vi "Get Element.vi"(8 "error in":errorcluster, 10 "element name":string, 11 "cluster in":variant) -> (0 "error out":errorcluster, 2 "element":variant, 3 "cluster out":variant)   [LabVIEW 2020, in "PV Access.lvlib" / "PV Data.lvlib"]
uses:
  PV Data.lvlib
  <userlib>/_OpenG.lib/lvdata/lvdata.llb/openg_variant.lvlib
  <userlib>/_OpenG.lib/error/error.llb/openg_error.lvlib
  Error Codes.ctl
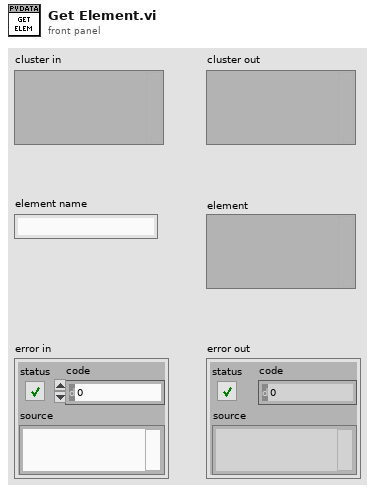
[diagram p1: front panel]
types:
  T1 = typedef "PV Access.lvlib/PV Data.lvlib/Error Codes.ctl" = i32
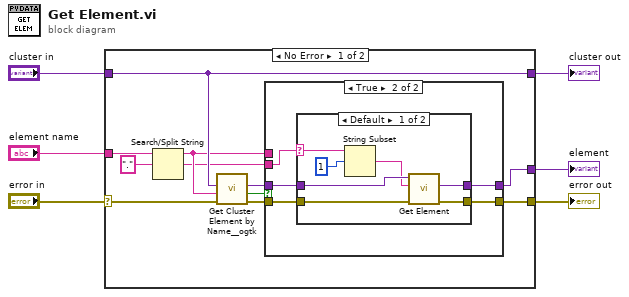
[diagram p0: block diagram]
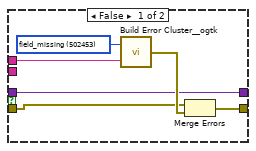
[diagram p2: hidden frame]
diagram:
  n1 = case shown="No Error" "error in" {
    selector: "error in" -> [w15 w39]
    tunnel: [w7 w39] -> w2
    tunnel: "element name" -> [w17 _]
    tunnel: "cluster in" -> [w14 w38]
    tunnel: [w14 w38] -> w3
    tunnel: [w8 _] -> w1
    frame No Error {
      n2 = Search/Split String(string=w17, search string/char (-)=".") -> (substring before match=w10:string, match + rest of string=w9:string)  [unwired: 1 in, 1 out]
      n3 = call <userlib>:"Get Cluster Element by Name__ogtk.vi"("error in (no error)"=w15, "Element Name"=w10, "Cluster"=w14) -> ("error out"=w13:errorcluster, "found?"=w12:bool, "VElement"=w11:variant)  [unwired: 6 in]
      n4 = case shown="True" w12 {
        tunnel: [w19 w24] -> w7
        tunnel: w13 -> [w20 w27]
        tunnel: w10 -> [w22 _]
        tunnel: w11 -> [w18 w26]
        tunnel: [w18 w25] -> w8
        tunnel: w9 -> [_ w28]
        frame False {
          w23 = T1 502453 items=["unspecified"=502450, "interrupted"=502451, "timeout"=502452, "field_missing"=502453, "cannot_convert_value"=502454, "type_mismatch"=502455] ("Ring")
          n5 = call <userlib>:"Build Error Cluster__ogtk.vi"("String to Prepend to source (\"\")"=w22, "code"=w23) -> ("error out"=w21:errorcluster)
          n6 = Merge Errors(w20, w21) -> (w19:errorcluster)
        }
        frame True {
          n7 = case shown="Default" w28 {
            selector: w28 -> [w34 _]
            tunnel: w27 -> [w33 w36]
            tunnel: w26 -> [w32 w37]
            tunnel: [w29 w37] -> w25
            tunnel: [w30 w36] -> w24
            frame Default {
              n8 = String Subset(string=w34, offset (0)=1) -> (substring=w31:string)  [unwired: 1 in]
              n9 = call "Get Element.vi"("error in"=w33, "element name"=w31, "cluster in"=w32) -> ("error out"=w30:errorcluster, "element"=w29:variant)  [unwired: 6 in, 1 out]
            }
            frame "" {
            }
          }
        }
      }
    }
    frame Error {
    }
  }
  "error out" <- w2
  "cluster out" <- w3
  "element" <- w1
